vi "G#Object_GetCommonQueueName.vi"(5 "error in (no error)":errorcluster) -> (14 "queue name":string, 19 "error out":errorcluster)   [LabVIEW 2017, in "G#Object.lvclass"]
doc: "Returns the name of the G# common queue. This is depended on the lib containing the G#Object class. Especially to avoid naming conflict with packed libraries."
uses:
  G#Object.lvclass
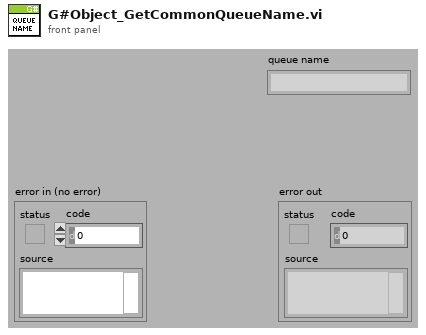
[diagram p1: front panel]
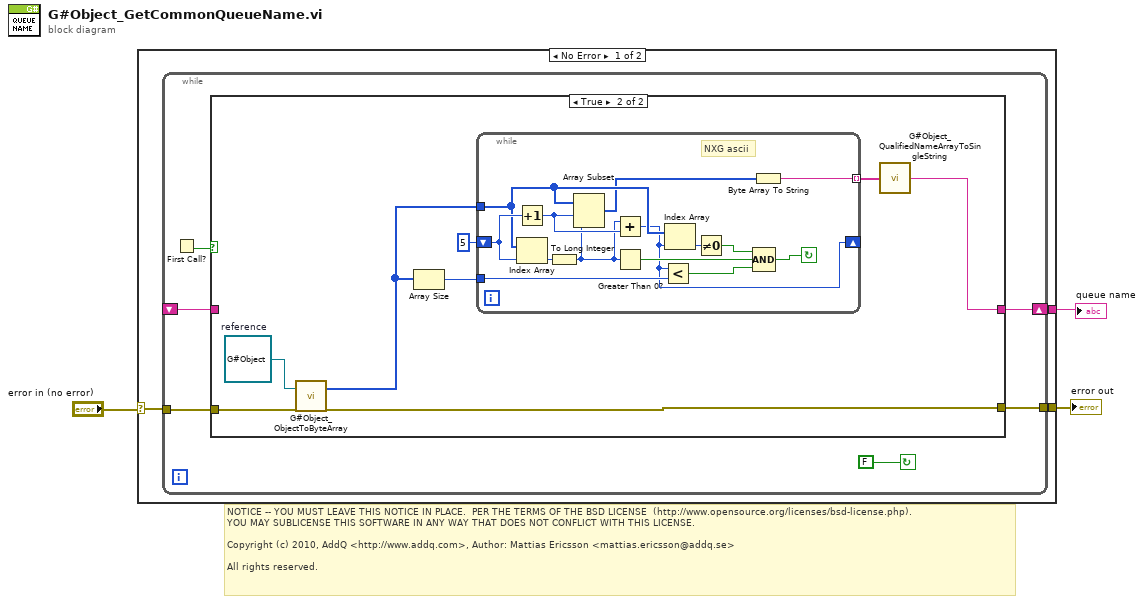
[diagram p0: block diagram]
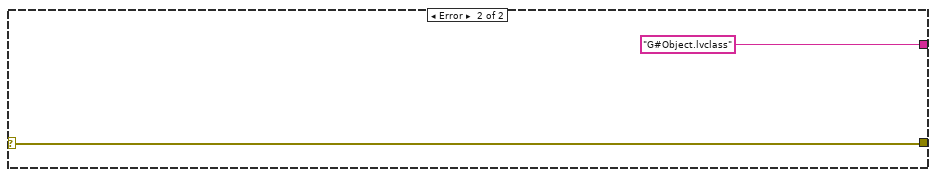
[diagram p3: hidden frame]
diagram:
  # "NOTICE -- YOU MUST LEAVE THIS NOTICE IN PLACE.  PER THE TERMS OF THE BSD LICENSE  (http://www.opensource.org/licenses/bsd-license.php).\nYOU MAY SUBLICENSE THIS SOFTWARE IN ANY WAY THAT DOES NOT CONFLICT WITH THIS LICENSE.\n\nCopyright (c) 2010, AddQ <http://www.addq.com>, Author: Mattias Ericsson <mattias.ericsson@addq.se>\n\nAll rights reserved."
  n1 = case shown="No Error" "error in (no error)" {
    selector: "error in (no error)" -> [w4 w38]
    tunnel: [w6 w38] -> w3
    tunnel: [w5 "G#Object.lvclass" ("Fully Qualified String")] -> w2
    frame No Error {
      n2 = while {
        tunnel: w4 -> [w12]
        tunnel: [w11] -> w6
        shift-right: [w10] -> w5
        shift-left: _ -> [w7]
        stop <- FALSE continue-if-true
        n3 = First Call?() -> (First Call?: T/F=w8:bool)
        n4 = case shown="True" w8 {
          tunnel: w12 -> [w14 w18]
          tunnel: [w14 w17] -> w11
          tunnel: [w13 w15] -> w10
          tunnel: w7 -> [w13 _]
          frame False {
          }
          frame True {
            w19 = refnum<class "G#Object.lvclass"> refnum  # reference
            n5 = call "G#Object_ObjectToByteArray.vi"("reference"=w19, "error in (no error)"=w18) -> ("unsigned byte array"=w20:u8[], "error out"=w17:errorcluster)  [unwired: 16 in]
            n6 = Array Size(array=w20) -> (size(s)=w21:i32)
            n7 = while {
              shift-right: [w27] -> _
              shift-left: 5 -> [w33]
              tunnel: w21 -> [w34]
              tunnel: [w29] -> w16 mode=indexing
              tunnel: w20 -> [w30]
              stop <- w25 continue-if-true
              # "NXG ascii"
              n8 = Increment(x=w33) -> (x+1=w28:i32)
              n9 = Index Array(array=w30, index=w33) -> (element=w24:u8)
              n10 = To Long Integer(number=w24) -> (32bit integer=w23:i32)
              n11 = Array Subset(array=w30, index=w28, length=w23) -> (w26:u8[])
              n12 = Add(x=w23, y=w28) -> (x+y=w27:i32)
              n13 = Greater Than 0?(x=w23) -> (x > 0?=w36:bool)
              n14 = Less?(x=w27, y=w34) -> (x < y?=w35:bool)
              n15 = Index Array(array=w30, index=w27) -> (element=w32:u8)
              n16 = Not Equal To 0?(x=w32) -> (x != 0?=w31:bool)
              n17 = Byte Array To String(unsigned byte array=w26) -> (string=w29:string)
              n18 = Compound Arithmetic op=AND(w31, w36, w35) -> (w25:bool)
            }
            n19 = call "G#Object_QualifiedNameArrayToSingleString.vi"("Fully Qualified Array"=w16) -> ("Fully Qualified String"=w15:string)
          }
        }
      }
    }
    frame Error {
    }
  }
  "error out" <- w3
  "queue name" <- w2
